vi "Write Actor.vi"(10 "Actor":refnum<data-value>, 11 "TEMPLATE Actor in":refnum<class "TEMPLATE Actor.lvclass">) -> (3 "TEMPLATE Actor out":refnum<class "TEMPLATE Actor.lvclass">)   [LabVIEW 2020, in "_Template.lvlib" / "Templates.lvlib" / "TEMPLATE jettl Actor.lvlib" / "TEMPLATE Actor.lvlib" / "TEMPLATE Actor.lvclass"]
uses:
  TEMPLATE Actor.lvclass
  TEMPLATE Actor.lvclass/TEMPLATE Actor.ctl
  jettl/jettl/jettl.lvlib
  jettl/jettl/Actor/Actor.lvclass
  jettl/jettl/Msg/Msg.lvclass
  jettl/jettl/Msgs.ctl
  jettl/jettl/Layer.ctl
  jettl/jettl/Refs/Refs.lvclass
  jettl/jettl/Actor.ctl
panel:
  # "This front panel should not be manipulated."
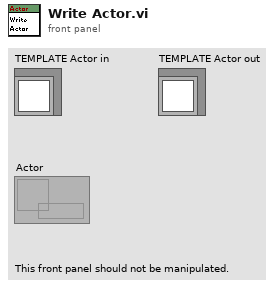
[diagram p1: front panel]
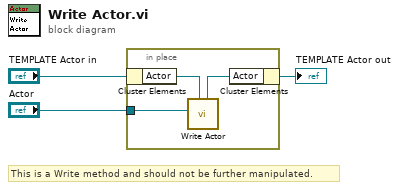
[diagram p0: block diagram]
diagram:
  # "This is a Write method and should not be further manipulated."
  n1 = in-place {
    in-place-border: "Actor" -> [w4]
    n2 = in-place-cluster #1("TEMPLATE Actor in") -> ("Actor"=w6:refnum<data-value>)
    n3 = call "Write Actor.vi"("Actor in"=w6, "Actor"=w4) -> ("Actor out"=w5:refnum<data-value>)  [unwired: 9 in]
    n4 = in-place-cluster #1("Actor"=w5) -> (→"TEMPLATE Actor out":refnum<class "TEMPLATE Actor.lvclass">)
  }
